vi "OpenPreprocSession.vi"(8 "error in (no error)":errorcluster, 10 "Python version":string="3.6", 11 "Python in":refnum<class "Python.lvclass">) -> (0 "error out":errorcluster, 3 "Python out":refnum<class "Python.lvclass">)   [LabVIEW 2020, in "Python.lvclass"]
uses:
  Python.lvclass
  Python.lvclass/Python.ctl
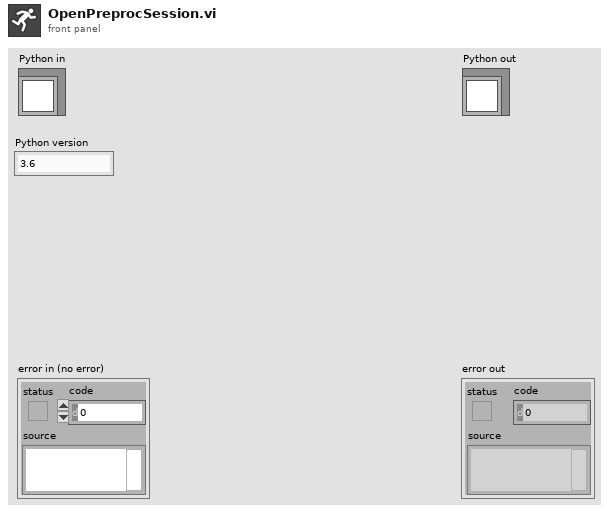
[diagram p1: front panel]
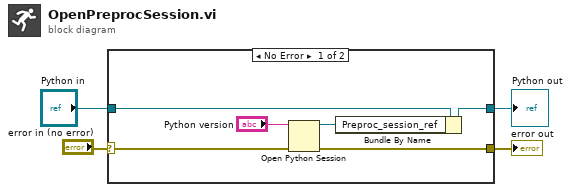
[diagram p0: block diagram]
diagram:
  n1 = case shown="No Error" "error in (no error)" {
    selector: "error in (no error)" -> [w8 w12]
    tunnel: [w7 w12] -> w3
    tunnel: [w6 w11] -> w1
    tunnel: "Python in" -> [w10 w11]
    frame No Error {
      n2 = Open Python Session(python version="Python version", 3:w8) -> (session out=w5:refnum<k35>, error out=w7:errorcluster)  [unwired: 1 in]
      n3 = Bundle By Name(cluster=w10, "Preproc_session_ref"=w5) -> (w6:refnum<class "Python.lvclass">)
    }
    frame Error {
    }
  }
  "error out" <- w3
  "Python out" <- w1
